vi "TableReceiverTactic.vi"(7 "Firstcall?":bool=TRUE, 8 "error in (no error)":errorcluster, 9 "Game in":refnum<class "Game.lvclass">, 10 "Robot":refnum<class "Robot.lvclass">, 11 "TableReceiverTactic in":refnum<class "TableReceiverTactic.lvclass">) -> (0 "error out":errorcluster, 2 "Robot out":refnum<class "Robot.lvclass">, 3 "TableReceiverTactic out":refnum<class "TableReceiverTactic.lvclass">)   [LabVIEW 2023, in "TableReceiverTactic.lvclass"]
uses:
  TableReceiverTactic.lvclass
  Robot_class/Robot.lvclass
  Game_class/Game.lvclass
  Robot_class/tactics.ctl
  Tactic_class/Tactic.lvclass/Tactic.ctl
  Game_class/Game.lvclass/Game.ctl
  Skillbook_class/Skillbook.lvclass/Skillbook.ctl
  Robot_class/Robot.lvclass/Robot.ctl
  TableReceiverTactic.lvclass/TableReceiverTactic.ctl
  Skillbook_class/Read TableReceiverGoToSkill.vi
  Game_class/Read Utilities.lvclass.vi
  Game_class/Read BallRef.vi
  Skillbook_class/Read HaltSkill.vi
  Robot_class/Write dest_orientation.vi
  Game_class/Read OffensiveTeam.vi
  Tactic_class/Read Skillbook.vi
  Write States.vi
  Robot_class/Write tactic.vi
  Utilities_class/Utilities.lvclass
  Ally_class/Ally.lvclass
  Ball_class/Ball.lvclass
  Skillbook_class/Skillbook.lvclass
  TableReceiverGoToSkill_class/TableReceiverGoToSkill.lvclass
  HaltSkill_class/HaltSkill.lvclass
panel:
  out "x .or. y?":bool
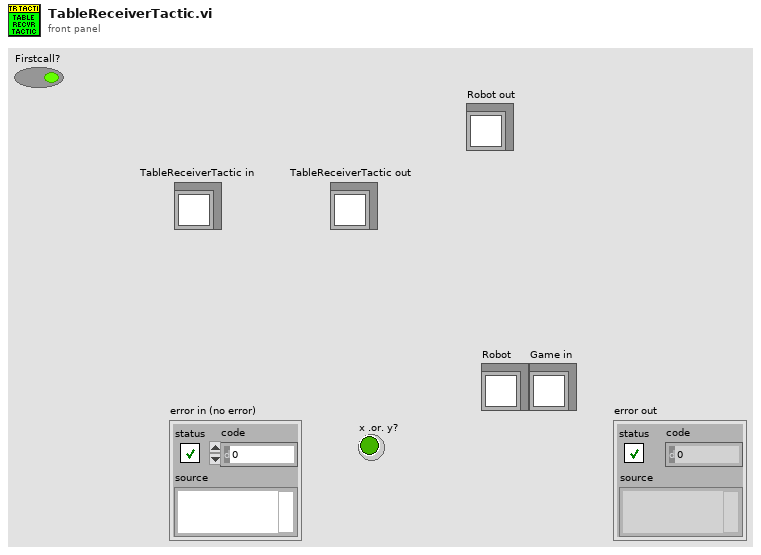
[diagram p1: front panel]
types:
  T1 = typedef "tactics.ctl" = enum16{"ReceivePassInFuturePoint", "Roller", "PrepareRollToPassRollerGoTo", "PrepareRollToPassReceiverGoTo", "WaitRoll", "PositionToRoll", "PenaltyAttacker", "PassObserver", "PenaltyDefense", "TableReceiverTactic", "Test", "DefendGoal", "Marker", "FollowAttacker", "DefendArea", "Shoot", "AttackerAimGoal", "AttackerBallOutOfField", "AttackerBlock", "AttackerStop", "Duelist", "Halt", "ZigZag", "GoTo", "Timeout", "KickToPassReceiver", "PositionToReceivePass", "DefendAreaVSS", "DefendGoalVSS", "KickVSS", "AttackVSS", "DispBallVSS", "PenaltyAttackVSS", "WaitPass"}
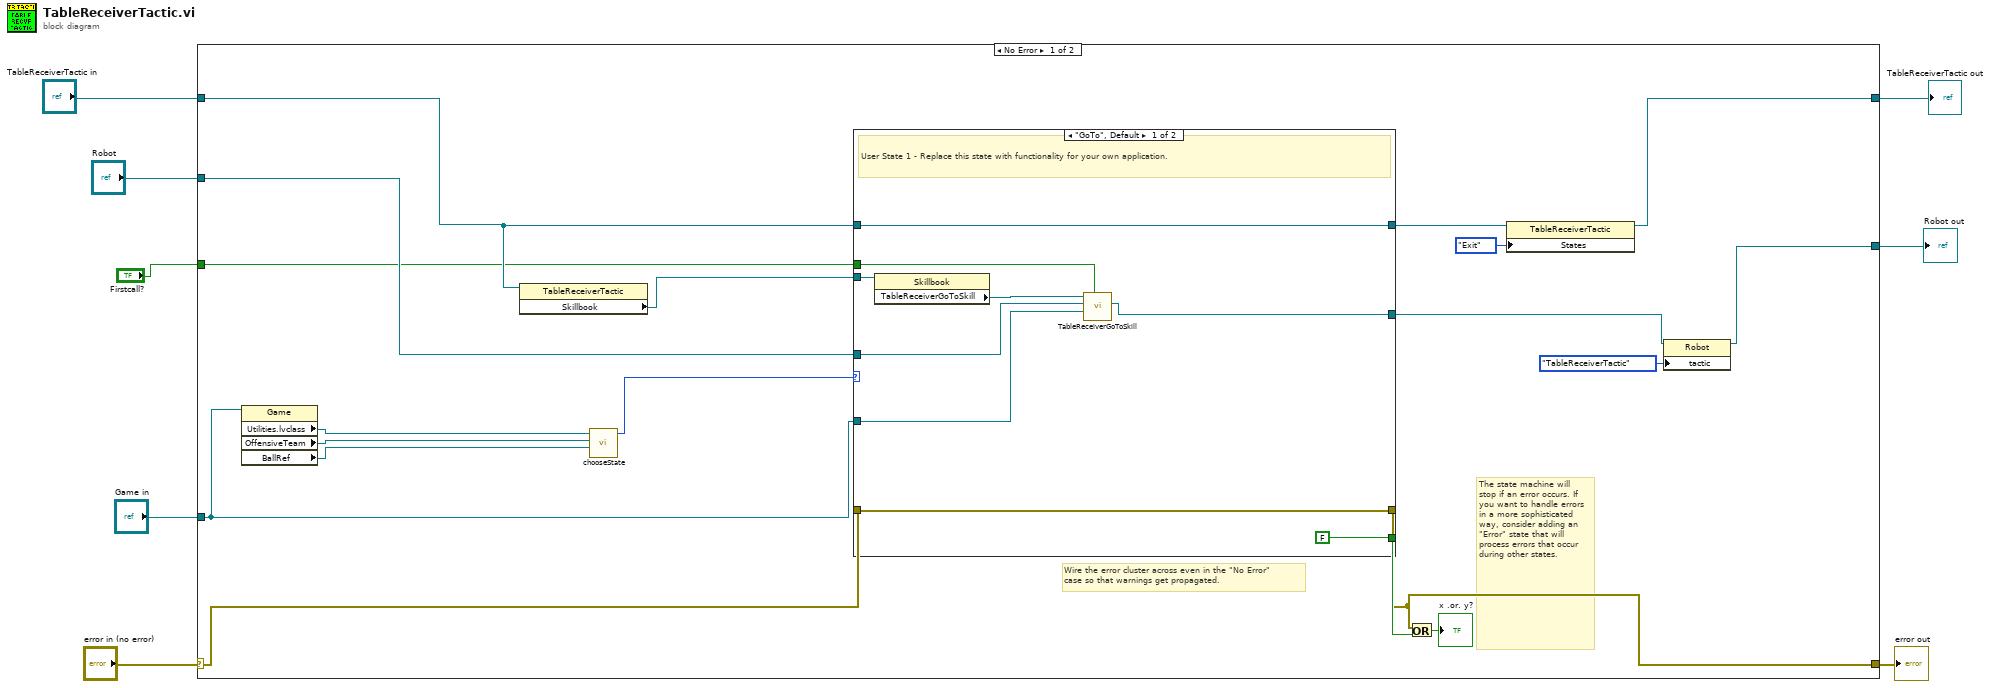
[diagram p0: block diagram]
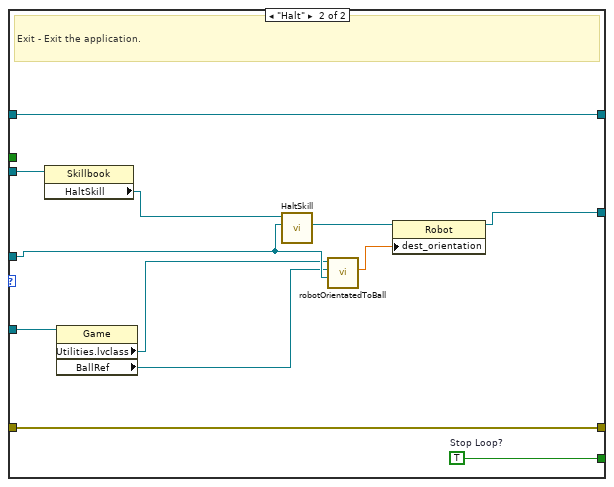
[diagram p2: hidden frame]
diagram:
  n1 = case shown="No Error" "error in (no error)" {
    selector: "error in (no error)" -> [w23 w51]
    tunnel: [w22 w51] -> w7
    tunnel: [w19 w50] -> w2
    tunnel: "TableReceiverTactic in" -> [w21 w50]
    tunnel: "Robot" -> [w20 w49]
    tunnel: "Game in" -> [w14 _]
    tunnel: [w17 w49] -> w4
    tunnel: "Firstcall?" -> [w10 _]
    frame No Error {
      # "The state machine will stop if an error occurs. If you want to handle errors in a more sophisticated way, consider adding an \"Error\" state that will process errors that occur during other states."
      # "Wire the error cluster across even in the \"No Error\"\ncase so that warnings get propagated."
      n2 = property class="Game"(reference=w14) -> ("Utilities.lvclass"=w16:refnum<class "Utilities.lvclass">, "OffensiveTeam"=w15:refnum<class "Ally.lvclass">, "BallRef"=w9:refnum<class "Ball.lvclass">)  [unwired: 1 in, 2 out]
      n3 = property class="TableReceiverTactic"(reference=w21) -> ("Skillbook"=w25:refnum<class "Skillbook.lvclass">)  [unwired: 1 in, 2 out]
      n4 = call "chooseState.vi"("BallRef"=w9, "OffensiveTeam"=w15, "Utilities in"=w16) -> ("States"=w12:enum16{"Halt", "Exit", "GoTo"})  [unwired: 8 in]
      n5 = case shown="\"GoTo\", Default" w12 {
        tunnel: [FALSE ("Stop Loop?") w48] -> w27
        tunnel: w23 -> [w35 w47]
        tunnel: [w35 w47] -> w22
        tunnel: w25 -> [w34 w45]
        tunnel: w20 -> [w30 w40]
        tunnel: [w31 w42] -> w18
        tunnel: [w33 w46] -> w24
        tunnel: w21 -> [w33 w46]
        tunnel: w14 -> [w29 w39]
        tunnel: w10 -> [w28 _]
        frame "GoTo", Default {
          # "User State 1 - Replace this state with functionality for your own application."
          n6 = property class="Skillbook"(reference=w34) -> ("TableReceiverGoToSkill"=w32:refnum<class "TableReceiverGoToSkill.lvclass">)  [unwired: 1 in, 2 out]
          n7 = call "TableReceiverGoToSkill.vi"("Firstcall?"=w28, "Game"=w29, "Robot in"=w30, "TableReceiverGoToSkill in"=w32) -> ("Robot out"=w31:refnum<class "Robot.lvclass">)  [unwired: 5 in, 2 out]
        }
        frame "Halt" {
          w48 = TRUE  # Stop Loop?
          # "Exit - Exit the application."
          n8 = property class="Skillbook"(reference=w45) -> ("HaltSkill"=w44:refnum<class "HaltSkill.lvclass">)  [unwired: 1 in, 2 out]
          n9 = property class="Game"(reference=w39) -> ("Utilities.lvclass"=w37:refnum<class "Utilities.lvclass">, "BallRef"=w38:refnum<class "Ball.lvclass">)  [unwired: 1 in, 2 out]
          n10 = call-dynamic "HaltSkill.vi"("Robot"=w40, "HaltSkill in"=w44) -> ("Robot out"=w43:refnum<class "Robot.lvclass">)  [unwired: 7 in, 2 out]
          n11 = call "robotOrientatedToBall.vi"("Robot"=w40, "BallRef"=w38, "Utilities in"=w37) -> ("Orientation"=w41:dbl)  [unwired: 6 in, 2 out]
          n12 = property class="Robot"(reference=w43, "dest_orientation"=w41) -> (reference out=w42:refnum<class "Robot.lvclass">)  [unwired: 1 in, 1 out]
        }
      }
      n13 = Or(x=w22, y=w27) -> (x .or. y?=→"x .or. y?":bool)
      n14 = property class="TableReceiverTactic"(reference=w24, "States"=enum16{"Halt", "Exit", "GoTo"}."Exit") -> (reference out=w19:refnum<class "TableReceiverTactic.lvclass">)  [unwired: 1 in, 1 out]
      n15 = property class="Robot"(reference=w18, "tactic"=tactics."TableReceiverTactic") -> (reference out=w17:refnum<class "Robot.lvclass">)  [unwired: 1 in, 1 out]
    }
    frame Error {
    }
  }
  "error out" <- w7
  "Robot out" <- w4
  "TableReceiverTactic out" <- w2
